vi "TestExec.Add Data Folder Items to Menu.vi"(6 "Working Dirs":T1[](array[typedef]), 7 "Enabled":bool, 11 "menu ref":refnum<k9>) -> (0 "error out":errorcluster)   [LabVIEW 2018]
uses:
  Common/Utils/TestExec/TestExec.WorkingDir.ctl
  <vilib>/KATE/Menu/Menu Utils.lvlib
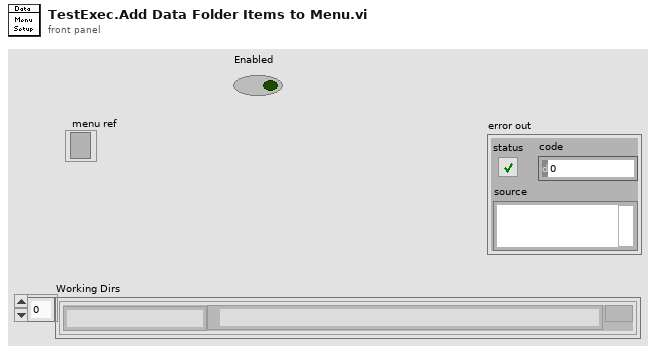
[diagram p1: front panel]
types:
  T1 = typedef "TestExec.WorkingDir.ctl" = cluster{"Name":string, "Path":path}
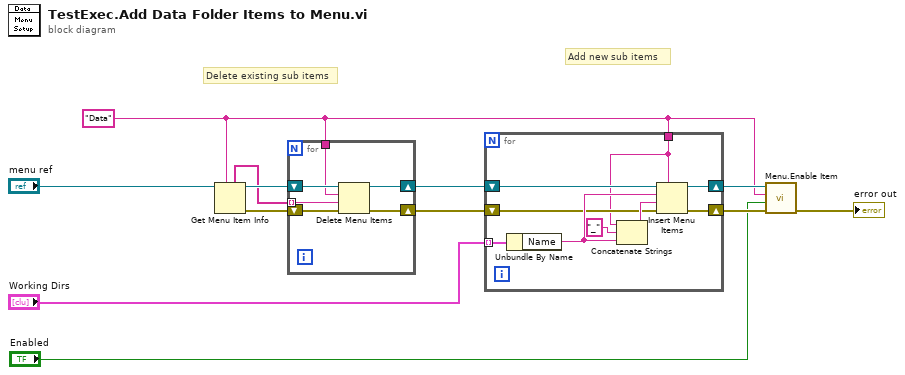
[diagram p0: block diagram]
diagram:
  w2 = "Data"
  # "Add new sub items"
  # "Delete existing sub items"
  n1 = Get Menu Item Info(7:w2, 11:"menu ref") -> (0:w9:errorcluster, 3:w11:refnum<k9>, 5:w10:string[])  [unwired: 1 in, 4 out]
  n2 = for {
    shift-right: [w18] -> w8
    shift-left: w11 -> [w17]
    tunnel: w2 -> [w16]
    tunnel: w10 -> [w15] mode=indexing
    shift-right: [w13] -> w6
    shift-left: w9 -> [w14]
    n3 = Delete Menu Items(6:w14, 7:w15, 8:w16, 9:w17) -> (0:w13:errorcluster, 3:w18:refnum<k9>)
  }
  n4 = for {
    shift-right: [w23] -> w7
    shift-left: w8 -> [w24]
    shift-right: [w21] -> w5
    shift-left: w6 -> [w22]
    tunnel: "Working Dirs" -> [w20] mode=indexing
    tunnel: w2 -> [w19]
    n5 = Unbundle By Name(w20) -> ("Name"=w26:string)
    n6 = Concatenate Strings(w19, "_", w26) -> (w27:string)
    n7 = Insert Menu Items(5:w19, 6:w22, 7:w27, 8:w26, 9:w24) -> (0:w21:errorcluster, 3:w23:refnum<k9>)  [unwired: 1 in, 1 out]
  }
  n8 = call <vilib>:"Menu.Enable Item.vi"("error in"=w5, "Enable"="Enabled", "Tag"=w2, "Menu Ref"=w7) -> ("error out"=→"error out":errorcluster)  [unwired: 6 in, 1 out]
